vi "LogError.vi"(8 "Error In":errorcluster, 11 "Path":path) -> (0 "Error Out":errorcluster, 3 "path":path)   [LabVIEW 2015]
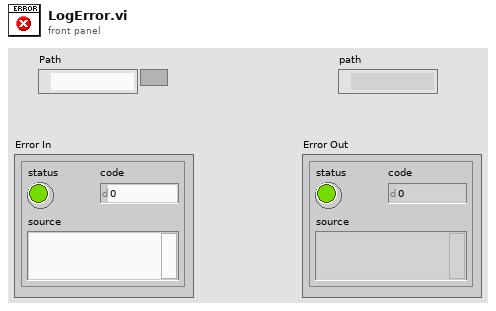
[diagram p1: front panel]
types:
  T1 = enum16{"open", "replace", "create", "open or create", "replace or create", "replace or create with confirmation"}
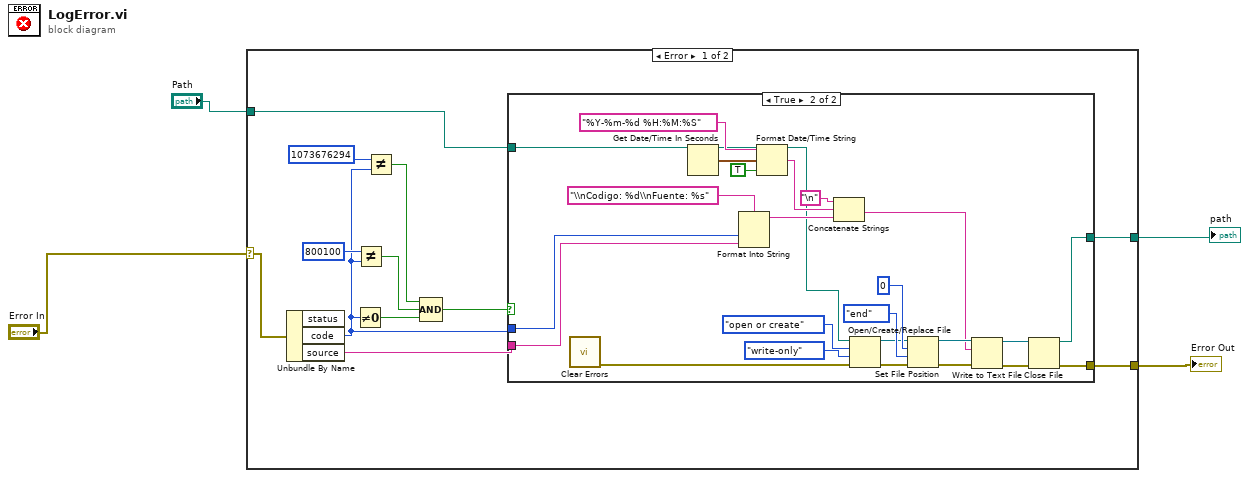
[diagram p0: block diagram]
diagram:
  n1 = case shown="Error" "Error In" {
    selector: "Error In" -> [w5 w43]
    tunnel: [w15 w43] -> w4
    tunnel: [w11 w42] -> w3
    tunnel: "Path" -> [w6 w42]
    frame Error {
      n2 = Unbundle By Name(w5) -> ("code"=w12:i32, "source"=w16:string)  [unwired: 1 out]
      n3 = Not Equal To 0?(x=w12) -> (x != 0?=w8:bool)
      n4 = Not Equal?(x=800100, y=w12) -> (x != y?=w9:bool)
      n5 = Not Equal?(x=1073676294, y=w12) -> (x != y?=w10:bool)
      n6 = Compound Arithmetic op=AND(w10, w9, w8) -> (w7:bool)
      n7 = case shown="True" w7 {
        tunnel: w16 -> [_ w40]
        tunnel: [_ w21] -> w15
        tunnel: w12 -> [_ w33]
        tunnel: w6 -> [w17 w20]
        tunnel: [w17 w19] -> w11
        frame False {
        }
        frame True {
          n8 = call <vilib>:"Clear Errors.vi"() -> ("error out"=w22:errorcluster)  [unwired: 6 in, 1 out]
          n9 = Get Date/Time In Seconds() -> (seconds since 1Jan1904=w38:timestamp)
          n10 = Format Into String(format string="\\nCodigo: %d\\nFuente: %s", w33, w40) -> (resulting string=w39:string)  [unwired: 2 in, 1 out]
          n11 = Format Date/Time String(time format string (%c)="%Y-%m-%d %H:%M:%S", seconds (now)=w38, UTC format=TRUE) -> (date/time string=w35:string)
          n12 = Concatenate Strings("\n", w35, w39) -> (w18:string)
          n13 = Open/Create/Replace File(file path (use dialog)=w20, error in=w22, operation (0:open)=T1."open or create", access (0:read/write)=enum16{"read/write", "read-only", "write-only"}."write-only") -> (refnum out=w23:refnum<file>, error out=w30:errorcluster)  [unwired: 2 in, 1 out]
          n14 = Set File Position(offset (in bytes) (0)=i64 0, refnum=w23, from (0:start)=enum16{"start", "end", "current"}."end", error in=w30) -> (refnum out=w28:refnum<file>, error out=w29:errorcluster)
          n15 = Write to Text File(file (use dialog)=w28, text=w18, error in=w29) -> (refnum out=w31:refnum<file>, error out=w32:errorcluster)  [unwired: 1 in, 1 out]
          n16 = Close File(refnum=w31, error in=w32) -> (path=w19:path, error out=w21:errorcluster)
        }
      }
    }
    frame No Error {
    }
  }
  "Error Out" <- w4
  "path" <- w3
